vi "Breakup Version String.vi"(11 "Vers String":string) -> (3 "Substrings":string[](array[string]))   [LabVIEW 2020, in "LMH-LINX.lvlib"]
uses:
  LMH-LINX.lvlib
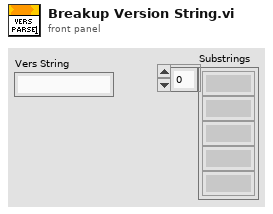
[diagram p1: front panel]
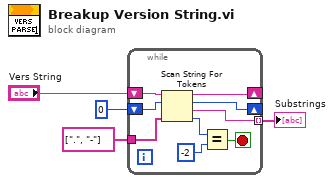
[diagram p0: block diagram]
diagram:
  n1 = while {
    shift-right: [w12] -> _
    shift-left: "Vers String" -> [w13]
    shift-right: [w10] -> _
    shift-left: 0 ("offset past token") -> [w11]
    tunnel: string[] [".", "-"] ("delimiters (\\s,\\t,\\r,\\n)") -> [w9]
    tunnel: [w5] -> w1 mode=indexing
    stop <- w6 stop-if-true
    n2 = Scan String For Tokens(6:w9, 8:w11, 9:w13) -> (0:w8:i32, 1:w5:string, 2:w10:i32, 3:w12:string)  [unwired: 3 in]
    n3 = Equal?(x=w8, y=-2 ("offset past token")) -> (x = y?=w6:bool)
  }
  "Substrings" <- w1
